vi "AOL Z Cal-Motor ctrl sequence.vi"(8 "error in (no error)":errorcluster, 10 "Wait before measurement (ms)":u32, 11 "Motor positions sequence":sgl[](array[numeric])) -> (0 "error out":errorcluster, 3 "Motor pos at max intensity":sgl)   [LabVIEW 2020]
uses:
  Globals/gl_Calibration globals.vi
  Global Variables/gl_Images.vi
  <vilib>/vision/NI_Vision_Development_Module.lvlib
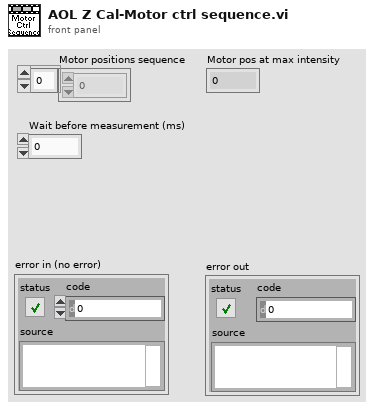
[diagram p1: front panel]
types:
  T1 = typedef "AOL Z cal process refs.ctl" = cluster{"This VI":refnum<vi>, "Abort (ind)":refnum<vi>, "Next (ind)":refnum<vi>, "Cancel":refnum<vi>, "Next":refnum<vi>, "Message":refnum<vi>, "Progress":refnum<vi>}
  T2 = typedef "Cal channel.ctl" = enum16{"Red Channel", "Green Channel"}
  T3 = typedef "IMAQ Image.ctl" = refnum<image>
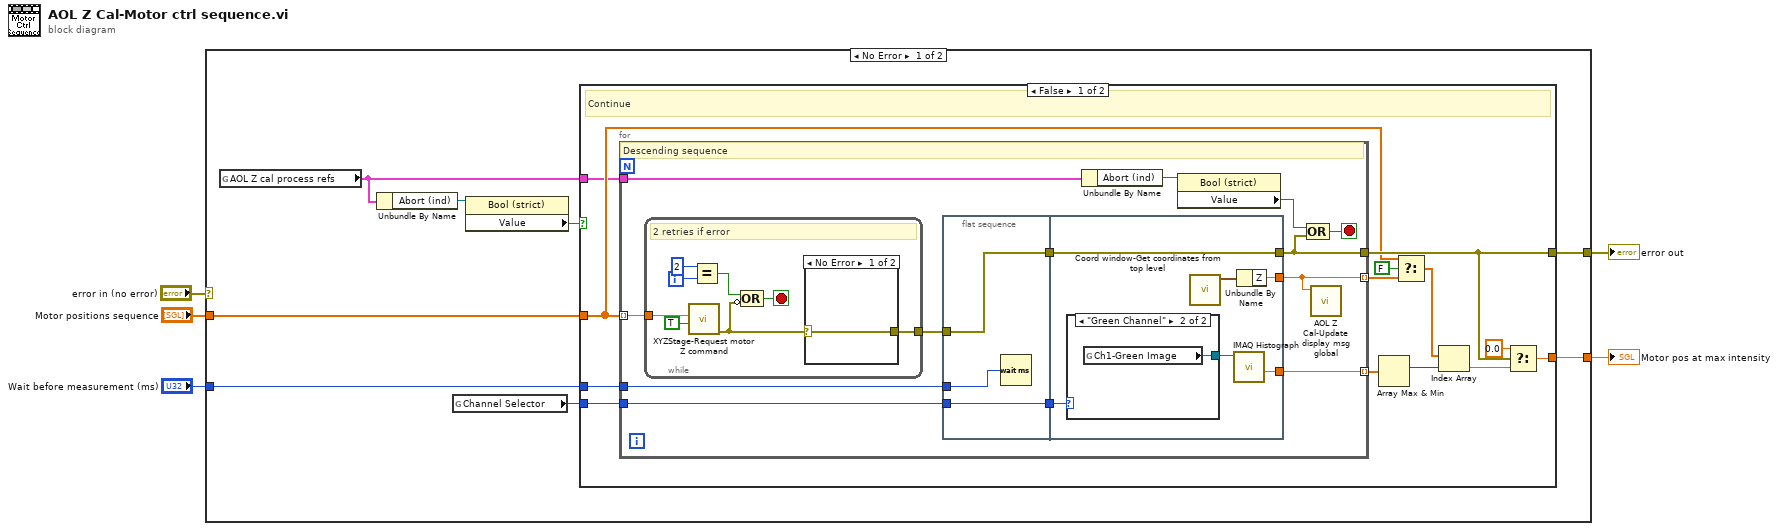
[diagram p0: block diagram]
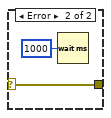
[diagram p2: hidden frame]
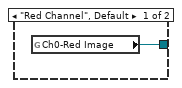
[diagram p3: hidden frame]
diagram:
  n1 = case shown="No Error" "error in (no error)" {
    selector: "error in (no error)" -> [_ w62]
    tunnel: "Wait before measurement (ms)" -> [w13 _]
    tunnel: [w11 w62] -> w4
    tunnel: [w12 _] -> w3
    tunnel: "Motor positions sequence" -> [w10 _]
    frame No Error {
      n2 = global read "gl_Calibration globals.vi" "AOL Z cal process refs"() -> (w8:T1)
      n3 = Unbundle By Name(w8) -> ("Abort (ind)"=w9:refnum<vi>)
      n4 = global read "gl_Calibration globals.vi" "Channel Selector"() -> (w6:T2)
      n5 = property class="Bool (strict)"(reference=w9) -> ("Value"=w7:bool)  [unwired: 1 in, 2 out]
      n6 = case shown="False" w7 {
        tunnel: w13 -> [w26 _]
        tunnel: w6 -> [w23 _]
        tunnel: [w22 _] -> w12
        tunnel: [w20 _] -> w11
        tunnel: w10 -> [w16 _]
        tunnel: w8 -> [w14 _]
        frame False {
          # "Continue"
          n7 = for {
            tunnel: w16 -> [w39] mode=indexing
            tunnel: w23 -> [w37]
            tunnel: [w36] -> w25 mode=indexing
            tunnel: [w30] -> w20
            tunnel: w26 -> [w33]
            tunnel: [w27] -> w18 mode=indexing
            tunnel: w14 -> [w31]
            stop <- w29 stop-if-true
            # "Descending sequence"
            n8 = while {
              tunnel: w39 -> [w47]
              tunnel: [w45] -> w34
              i -> [w44]
              stop <- w40 stop-if-true
              # "2 retries if error"
              n9 = call "XYZStage-Request motor Z command.vi"("Wait for acknowledge?"=TRUE, "Motor Z"=w47) -> ("error out"=w42:errorcluster)  [unwired: 7 in, 2 out]
              n10 = Equal?(x=2, y=w44) -> (x = y?=w41:bool)
              n11 = Compound Arithmetic op=OR(w41, invert w42) -> (w40:bool)
              n12 = case shown="No Error" w42 {
                selector: w42 -> [w48 w49]
                tunnel: [w48 w49] -> w45
                frame No Error {
                }
                frame Error {
                  n13 = Wait (ms)(milliseconds to wait=u32 1000) -> ()  [unwired: 1 out]
                }
              }
            }
            n14 = flat-sequence {
              tunnel: [w53] -> w38
              tunnel: w37 -> [w53]
              tunnel: [w52] -> w35
              tunnel: w34 -> [w52]
              tunnel: w33 -> [w51]
              tunnel: w38 -> [w59]
              tunnel: [w57] -> w36
              tunnel: [w56] -> w30
              tunnel: w35 -> [w56]
              tunnel: [w54] -> w27
              frame #0 {
                n15 = Wait (ms)(milliseconds to wait=w51) -> ()  [unwired: 1 out]
              }
              frame #1 {
                n16 = case shown="\"Green Channel\"" w59 {
                  tunnel: [w60 w61] -> w58
                  frame "Red Channel", Default {
                    n17 = global read "gl_Images.vi" "Ch0-Red Image"() -> (w60:T3)
                  }
                  frame "Green Channel" {
                    n18 = global read "gl_Images.vi" "Ch1-Green Image"() -> (w61:T3)
                  }
                }
                n19 = call "Coord window-Get coordinates from top level.vi"() -> ("Coordinates"=w55:cluster{"X":sgl, "Y":sgl, "Z":sgl})  [unwired: 11 in]
                n20 = call "IMAQ Histograph"("Image"=w58) -> ("Standard  Deviation"=w57:sgl)  [unwired: 7 in, 3 out]
                n21 = Unbundle By Name(w55) -> ("Z"=w54:sgl)
              }
            }
            n22 = Unbundle By Name(w31) -> ("Abort (ind)"=w32:refnum<vi>)
            n23 = property class="Bool (strict)"(reference=w32) -> ("Value"=w28:bool)  [unwired: 1 in, 2 out]
            n24 = Compound Arithmetic op=OR(w28, w30) -> (w29:bool)
            n25 = call "AOL Z Cal-Update display msg global.vi"("Motor Z"=w27) -> ()  [unwired: 11 in]
          }
          n26 = Array Max & Min(array=w25) -> (max index (indices)=w24:i32)  [unwired: 3 out]
          n27 = Select(t=w16, s=FALSE, f=w18) -> (s? t:f=w17:sgl[])
          n28 = Index Array(array=w17, index=w24) -> (element=w21:sgl)
          n29 = Select(t=sgl 0.0, s=w20, f=w21) -> (s? t:f=w22:sgl)
        }
        frame True {
          # "Cancelled by the user"
        }
      }
    }
    frame Error {
    }
  }
  "Motor pos at max intensity" <- w3
  "error out" <- w4
